vi "OP500ZP_MicroScan.vi"(6 "Dataout":string, 8 "Rev":string, 9 "SN":string, 10 "Oui":bool, 11 "str":string) -> (3 "Chaîne":string)   [LabVIEW 2020]
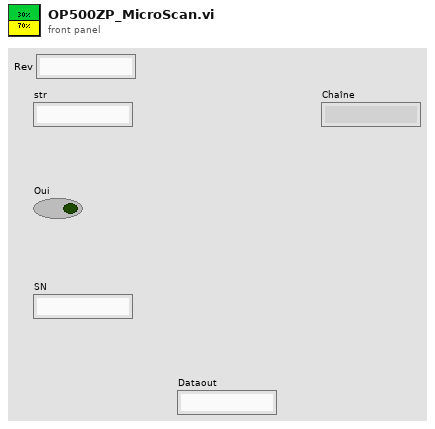
[diagram p1: front panel]
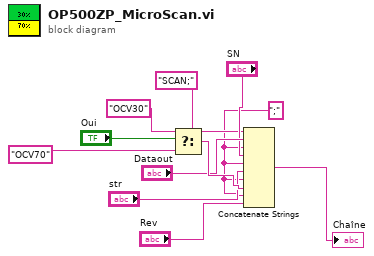
[diagram p0: block diagram]
diagram:
  w2 = ";" ("chaîne")
  n1 = Select ("Sélectionner")(t="OCV30" ("section"), s="Oui", f="OCV70" ("section")) -> (s? t:f=w10:string)
  n2 = Concatenate Strings("SCAN;" ("chaîne"), "Dataout", w2, "SN", w2, "str", w2, w10, w2, "Rev") -> (→"Chaîne":string)
